vi "IsIntEXT.vi"(4 "x":ext) -> (1 "Integer?":bool)   [LabVIEW 2017, in "GPComparison.lvlib"]
doc: "<B>Integer?</B> will be True if <B>x</B> is an integer.\n\nThis VI is inlined.\n\nSteen Schmidt\nGPower\n6/3 2013"
uses:
  GPComparison.lvlib
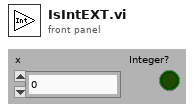
[diagram p1: front panel]
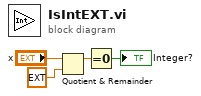
[diagram p0: block diagram]
diagram:
  n1 = Quotient & Remainder(x="x", y=ext 1.0) -> (x-y*floor(x/y)=w3:ext)  [unwired: 1 out]
  n2 = Equal To 0?(x=w3) -> (x = 0?=→"Integer?":bool)
